vi "Swerve_Cancel.vi"   [LabVIEW 2012]
uses:
  CLIB/CThread/Base/CThread Base - VI Reference.vi
  CLIB/CThread/Base/CThread Base - Cancel.vi
  CLIB/CThread/XNodes/referencenode/CThread VI Reference.xnode
  CLIB/CThread/XNodes/terminalnode/CThread VI Terminal Node.xnode
  CLIB/CThread/CThread.lvlib
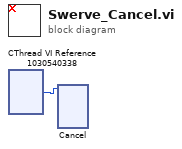
[diagram p0: block diagram]
diagram:
  n1 = xnode "CThread VI Reference 1030540338"() -> ("Swerve_Slave.vi"=w1:i32)
  n2 = xnode "Cancel"("CLIB VI Reference"=w1) -> ()  [unwired: 1 out]
